vi "Close.vi"(8 "error in (no error)":errorcluster, 11 "TesteractHAL_DigitalOutput_EthernetModbus In":refnum<class "TesteractHAL_DigitalOutput_EthernetModbus.lvclass">) -> (0 "error out":errorcluster, 3 "TesteractHAL_DigitalOutput_EthernetModbus Out":refnum<class "TesteractHAL_DigitalOutput_EthernetModbus.lvclass">)   [LabVIEW 2017, in "TesteractHAL_DigitalOutput_EthernetModbus.lvlib" / "TesteractHAL_DigitalOutput_EthernetModbus.lvclass"]
uses:
  TesteractHAL_DigitalOutput_EthernetModbus.lvclass
  C:/Program Files (x86)/Testeract/HWLib/HAL/Device/TesteractHAL_Device.lvlibp/TesteractHAL_Device.lvclass
  TesteractHAL_DigitalOutput_EthernetModbus.lvclass/TesteractHAL_DigitalOutput_EthernetModbus.ctl
  Program Files (x86)/Testeract/HWLib/HAL/Device/TesteractHAL_Device.lvlibp/ReadConnectionAlias.vi
  Program Files (x86)/Testeract/TCPConnectionManager/Testeract_TCPConnectionManager.lvlibp/Testeract_TCPConnectionManager.lvclass
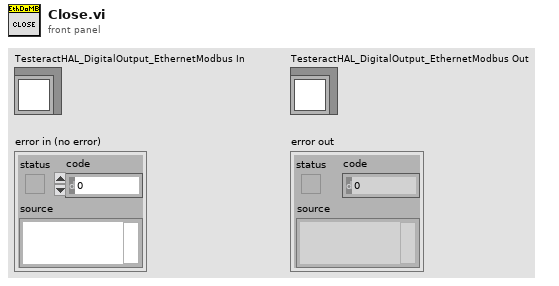
[diagram p1: front panel]
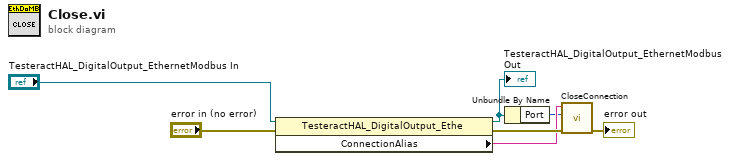
[diagram p0: block diagram]
diagram:
  n1 = property class="TesteractHAL_DigitalOutput_Ethe"(reference="TesteractHAL_DigitalOutput_EthernetModbus In", error in="error in (no error)") -> (reference out=w2:refnum<class "TesteractHAL_DigitalOutput_EthernetModbus.lvclass">, error out=w5:errorcluster, "ConnectionAlias"=w3:string)
  "TesteractHAL_DigitalOutput_EthernetModbus Out" <- w2
  n2 = Unbundle By Name(w2) -> ("Port"=w1:u16)
  n3 = call "CloseConnection.vi"("error in (no error)"=w5, "Port"=w1, "IPAddress"=w3) -> ("error out"=→"error out":errorcluster)  [unwired: 8 in]
